vi "Initialize Listbox.vi"(5 "remove":refnum<vi>, 7 "add":refnum<vi>, 8 "error in (no error)":errorcluster, 9 "Names":string[](array[string]), 10 "Listbox":refnum<vi>, 11 "Item Ref":T2=18446744073709551615 format="%.0x") -> (0 "error out":errorcluster, 3 "Listbox Refs":T1 {"Section Ref" format="%.0x"})   [LabVIEW 2019, in "FPGA Addon System Explorer.lvlib"]
uses:
  FPGA Addon System Explorer.lvlib
  <vilib>/NI VeriStand/Custom Device API/Custom Device Item Ref.ctl
  Listbox Cluster.ctl
  <vilib>/NI VeriStand/Custom Device API/Custom Device API.lvlib
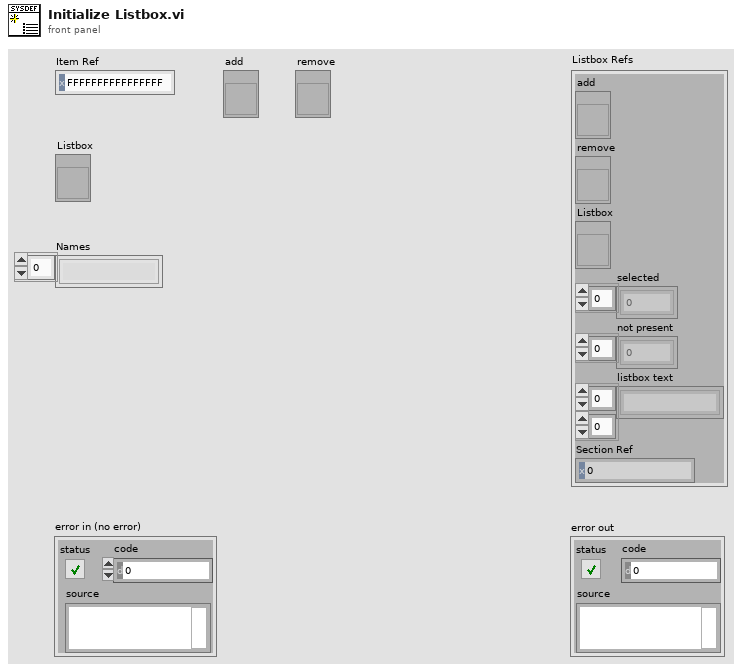
[diagram p1: front panel]
types:
  T1 = typedef "FPGA Addon System Explorer.lvlib/Listbox Cluster.ctl" = cluster{"add":refnum<vi>, "remove":refnum<vi>, "Listbox":refnum<vi>, "selected":i32[], "not present":i32[], "listbox text":string[][], "Section Ref":T2}
  T2 = typedef "Custom Device API.lvlib/Custom Device Item Ref.ctl" = u64
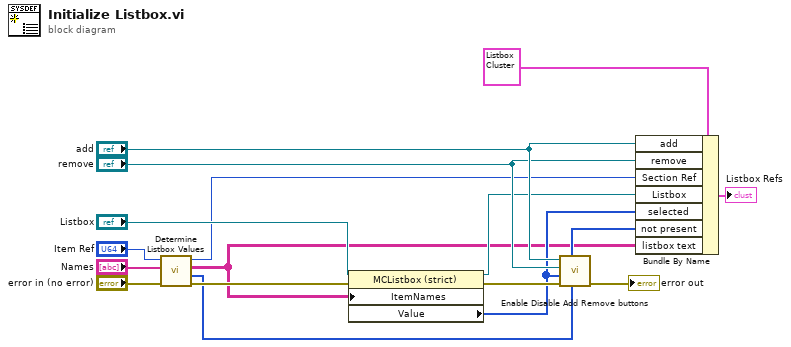
[diagram p0: block diagram]
diagram:
  n1 = call "Determine Listbox Values.vi"("error in (no error)"="error in (no error)", "List of Objects"="Names", "Section Ref in"="Item Ref") -> ("error out"=w12:errorcluster, "not present item indexes"=w3:i32[], "listbox text"=w2:string[][], "Section Ref out"=w6:T2)  [unwired: 5 in]
  n2 = property class="MCListbox (strict)"(reference="Listbox", error in=w12, "ItemNames"=w2) -> (reference out=w5:refnum<vi>, error out=w16:errorcluster, "Value"=w4:i32[])
  n3 = call "Enable Disable Add Remove buttons.vi"("not present item indexes"=w3, "error in (no error)"=w16, "selected items"=w4, "remove button"="remove", "add button"="add") -> ("error out"=→"error out":errorcluster)  [unwired: 6 in]
  n4 = Bundle By Name(cluster=T1 {"add"=refnum, "remove"=refnum, "Listbox"=refnum, "selected"=[], "not present"=[], "listbox text"=[], "Section Ref"=0}, "add"="add", "remove"="remove", "Section Ref"=w6, "Listbox"=w5, "selected"=w4, "not present"=w3, "listbox text"=w2) -> (→"Listbox Refs":T1)
